vi "MU Set Config.vi"(8 "error in (no error)":errorcluster, 9 "value":u32, 10 "configuration":u32, 11 "handle":u64) -> (0 "error out (no error)":errorcluster, 3 "function return":u32)   [LabVIEW 2017, in "MU_3SL_interface.lvlib"]
uses:
  MU_3SL_interface.lvlib
  lib/MU_3SL_interface.dll
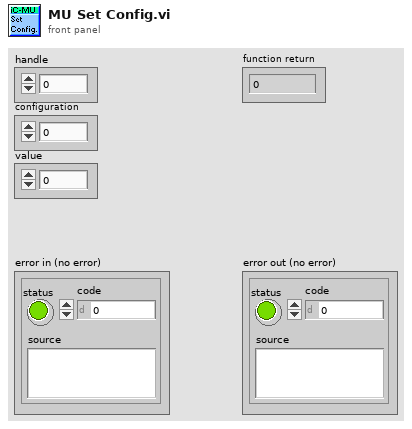
[diagram p1: front panel]
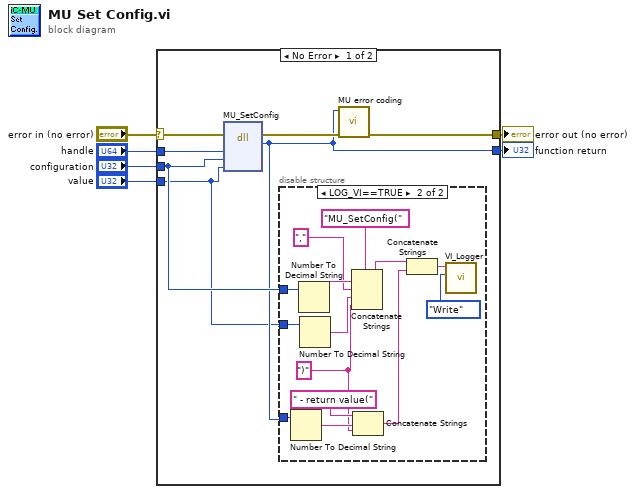
[diagram p0: block diagram]
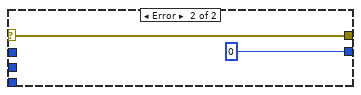
[diagram p3: hidden frame]
diagram:
  n1 = case shown="No Error" "error in (no error)" {
    selector: "error in (no error)" -> [w11 w29]
    tunnel: [w8 u32 0] -> w6
    tunnel: "handle" -> [w10 _]
    tunnel: "configuration" -> [w9 _]
    tunnel: "value" -> [w7 _]
    tunnel: [w12 w29] -> w2
    frame No Error {
      n2 = dll-call lib="C:/Users/bes/AppData/Roaming/work/mu_9so/icsubmodules/soft_mu_3sl_master/lv_interface/lib/MU_3SL_interface**.*" fn="MU_SetConfig"(error in=w11, "handle"=w10, "configuration"=w9, "value"=w7) -> (error out=w13:errorcluster, "return type"=w8:u32)  [unwired: 5 in, 1 out]
      n3 = disable-structure shown="LOG_VI==TRUE" {
        disable-tunnel: w8 -> [_ w25]
        disable-tunnel: w9 -> [_ w20]
        disable-tunnel: w7 -> [_ w17]
        frame condition #0 {
        }
        frame condition #1 (active) {
          w14 = ")" ("string")
          n4 = Number To Decimal String(number=w25) -> (decimal integer string=w24:string)  [unwired: 1 in]
          n5 = Number To Decimal String(number=w20) -> (decimal integer string=w19:string)  [unwired: 1 in]
          n6 = Number To Decimal String(number=w17) -> (decimal integer string=w16:string)  [unwired: 1 in]
          n7 = Concatenate Strings("MU_SetConfig(" ("Info in"), w19, "," ("string"), w16, w14) -> (w23:string)
          n8 = Concatenate Strings(" - return value(" ("string"), w24, w14) -> (w22:string)
          n9 = Concatenate Strings(w23, w22) -> (w21:string)
          n10 = call "VI_Logger.vi"("Action (Read)"=enum16{"Write", "Read"}."Write", "Info in"=w21) -> ()  [unwired: 8 in, 2 out]
        }
      }
      n11 = call "MU error coding.vi"("error in (no error)"=w13, "function return in"=w8) -> ("error out"=w12:errorcluster)  [unwired: 9 in]
    }
    frame Error {
    }
  }
  "function return" <- w6
  "error out (no error)" <- w2
